vi "Set Slot Programming Mode.vi"(8 "error in (no error)":errorcluster, 10 "Slot Programming Mode":T1, 11 "Refnum in":refnum<k20>) -> (0 "error out":errorcluster, 3 "Refnum out":refnum<k20>)   [LabVIEW 2019, in "Scan Engine Custom Device.lvlib"]
doc: "Apply new \"Slot Prgramming Mode\" property value."
uses:
  Scan Engine Custom Device.lvlib
  Type Defs/Slot Programming Mode.ctl
  <vilib>/nisyscfg/Save Changes (Hardware).vi
  <resource>/objmgr/nicriosae.rc
  <vilib>/nisyscfg/nisyscfg.lvlib
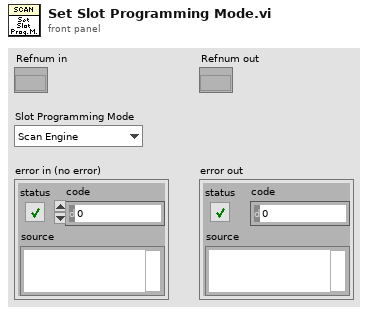
[diagram p1: front panel]
types:
  T1 = typedef "Scan Engine Custom Device.lvlib/Slot Programming Mode.ctl" = enum16{"Scan Engine", "LabVIEW FPGA", "NI-DAQmx", "Don't Modify"}
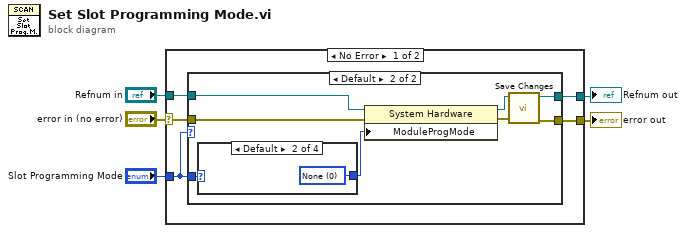
[diagram p0: block diagram]
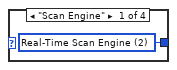
[diagram p3: hidden frame]
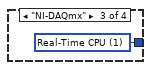
[diagram p4: hidden frame]
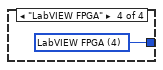
[diagram p5: hidden frame]
diagram:
  n1 = case shown="No Error" "error in (no error)" {
    selector: "error in (no error)" -> [w7 w25]
    tunnel: "Slot Programming Mode" -> [w6 _]
    tunnel: [w10 w26] -> w4
    tunnel: [w9 w25] -> w3
    tunnel: "Refnum in" -> [w8 w26]
    frame No Error {
      n2 = case shown="Default" w6 {
        tunnel: w6 -> [_ w19]
        tunnel: [w11 w18] -> w10
        tunnel: [w12 w17] -> w9
        tunnel: w8 -> [w11 w14]
        tunnel: w7 -> [w12 w13]
        frame "Don't Modify" {
        }
        frame Default {
          n3 = case shown="Default" w19 {
            tunnel: [w21 w22 w23 w24] -> w20
            frame "Scan Engine" {
              w21 = u32 2 items=["None"=0, "Real-Time CPU"=1, "Real-Time Scan Engine"=2, "LabVIEW FPGA"=4] ("Devices & Chassis:Bus Specific:cRIO Module Programming Mode")
            }
            frame Default {
              w22 = u32 0 items=["None"=0, "Real-Time CPU"=1, "Real-Time Scan Engine"=2, "LabVIEW FPGA"=4] ("Devices & Chassis:Bus Specific:cRIO Module Programming Mode")
            }
            frame "NI-DAQmx" {
              w23 = u32 1 items=["None"=0, "Real-Time CPU"=1, "Real-Time Scan Engine"=2, "LabVIEW FPGA"=4] ("Devices & Chassis:Bus Specific:cRIO Module Programming Mode")
            }
            frame "LabVIEW FPGA" {
              w24 = u32 4 items=["None"=0, "Real-Time CPU"=1, "Real-Time Scan Engine"=2, "LabVIEW FPGA"=4] ("Devices & Chassis:Bus Specific:cRIO Module Programming Mode")
            }
          }
          n4 = property class="System Hardware"(reference=w14, error in=w13, "ModuleProgMode"=w20) -> (reference out=w16:refnum<k20>, error out=w15:errorcluster)
          n5 = call-poly <vilib>:"Save Changes.vi"("error in (no error)"=w15, "Resource in"=w16) -> ("error out"=w17:errorcluster, "Resource out"=w18:refnum<k20>)  [unwired: 6 in, 2 out]
        }
      }
    }
    frame Error {
    }
  }
  "Refnum out" <- w4
  "error out" <- w3
